vi "Do.vi"(8 "error in (no error)":errorcluster, 10 "Actor in":refnum<class "Actor.lvclass">, 11 "Concrete Cancel SAM from Settings Model Msg in":refnum<class "Concrete Cancel SAM.lvclass">) -> (0 "error out":errorcluster, 2 "Actor out":refnum<class "Actor.lvclass">)   [LabVIEW 2015, in "Message Dialog Model.lvlib" / "Concrete Cancel SAM.lvclass"]
doc: "(<B>Filename</B>: Actor Framework.lvlib:Message.lvclass:Do.vi)\n\nDefines what a message does when it is received by an actor. Generally, a message instructs an actor to invoke one of its methods.\n\nBy default, this method does nothing. A child class must override it to define behavior. Create a child class by using the Actor Framework Message Maker dialog box."
uses:
  Concrete Cancel SAM.lvclass
  <vilib>/ActorFramework/Actor/Actor.lvclass
  Message Dialog Model/Message Dialog Model.lvclass
  Message Dialog Model/Message Dialog Model.lvclass/Message Dialog Model.ctl
  Settings Model/Settings Model Messages/Abstract Cancel SAM Msg/Abstract Cancel SAM Msg.lvclass
panel:
  # "NOTICE -- YOU MUST LEAVE THIS NOTICE IN PLACE.\n\nCopyright (c) 2015, LIANG LIU Shawn.Liu.cn@gmail.com\nAll rights reserved.\n\nRedistribution and use in source and binary forms, with or without modification, are permitted provided that the following conditions are met:\n-Redistributions of source code must retain the above copyright notice, this list of conditions and the following disclaimer.\n-Redistributions in binary form must reproduce the above copyright notice, this list of conditions and the following disclaimer in the documentation and/or other materials provided with the distribution.\n-Neither the name of the eLp nor the names of its contributors may be used to endorse or promote products derived from this software without specific prior written permission.\n\nTHIS SOFTWARE IS PROVIDED BY THE COPYRIGHT HOLDERS AND CONTRIBUTORS \"AS IS\" AND ANY EXPRESS OR IMPLIED WARRANTIES, INCLUDING, BUT NOT LIMITED TO, THE IMPLIED WARRANTIES OF MERCHANTABILITY AND FITNESS FOR A PARTICULAR PURPOSE ARE DISCLAIMED. IN NO EVENT SHALL THE COPYRIGHT HOLDER OR CONTRIBUTORS BE LIABLE FOR ANY DIRECT, INDIRECT, INCIDENTAL, SPECIAL, EXEMPLARY, OR CONSEQUENTIAL DAMAGES (INCLUDING, BUT NOT LIMITED TO, PROCUREMENT OF SUBSTITUTE GOODS OR SERVICES; LOSS OF USE, DATA, OR PROFITS; OR BUSINESS INTERRUPTION) HOWEVER CAUSED AND ON ANY THEORY OF LIABILITY, WHETHER IN CONTRACT, STRICT LIABILITY, OR TORT (INCLUDING NEGLIGENCE OR OTHERWISE) ARISING IN ANY WAY OUT OF THE USE OF THIS SOFTWARE, EVEN IF ADVISED OF THE POSSIBILITY OF SUCH DAMAGE."
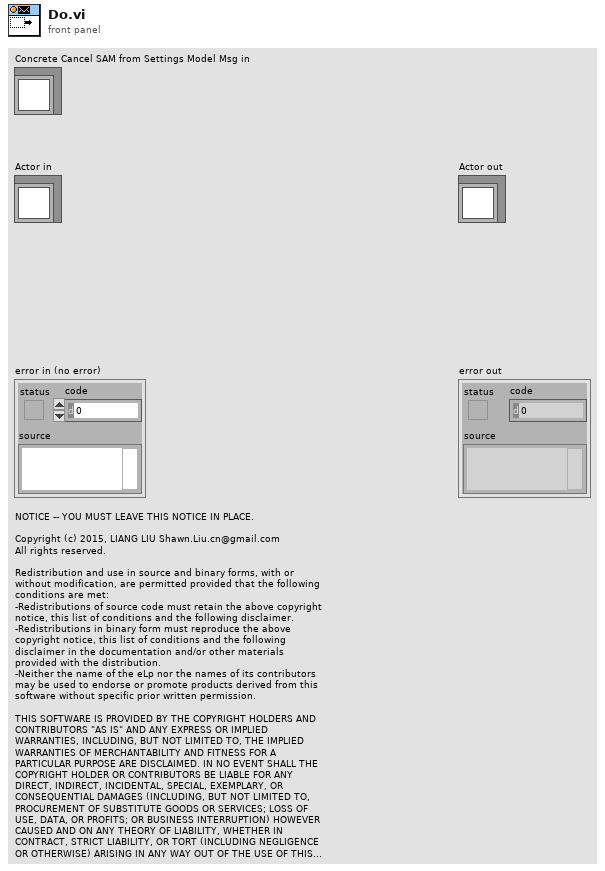
[diagram p1: front panel]
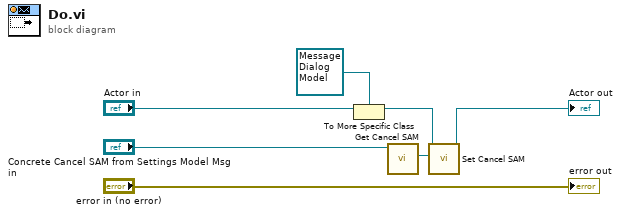
[diagram p0: block diagram]
diagram:
  n1 = To More Specific Class(target class=refnum<class "Message Dialog Model.lvclass"> refnum ("Message Model.lvlib:Message Model.lvclass"), reference="Actor in") -> (specific class reference=w4:refnum<class "Message Dialog Model.lvclass">)  [unwired: 1 in, 1 out]
  n2 = call "Get Cancel SAM.vi"("Abstract Cancel SAM Msg in"="Concrete Cancel SAM from Settings Model Msg in") -> ("Cancel SAM"=w2:refnum<class "Self-Addressed Msg.lvclass">)  [unwired: 9 in, 1 out]
  n3 = call "Set Cancel SAM.vi"("Cancel Msg"=w2, "Message Dialog Model in"=w4) -> ("Message Dialog Model out"=→"Actor out":refnum<class "Message Dialog Model.lvclass">)  [unwired: 9 in]
  "error out" <- "error in (no error)"
